vi "Channels.Inline.Write.Channel Block Descriptor (single).vi"(8 "error in (no error)":errorcluster, 10 "Values Array in":dbl[](array[numeric]), 11 "Channel Block Descriptor":T1) -> (0 "error out":errorcluster, 2 "Values Array out":dbl[](array[numeric]), 3 "Channel Block Descriptor dup":T1)   [LabVIEW 2016, in "VeriStand Data.lvlib"]
doc: "Writes the contents of <B>Values Array</B> to the memory location specified by <B>Channel Block Descriptor</B>."
uses:
  VeriStand Data.lvlib
  Typedefs/Typedefs.Block Descriptor.Channel Block.ctl
  Typedefs/Typedefs.Block Descriptor.ctl
  Memory Management/Memory Management.Handle Return.vi
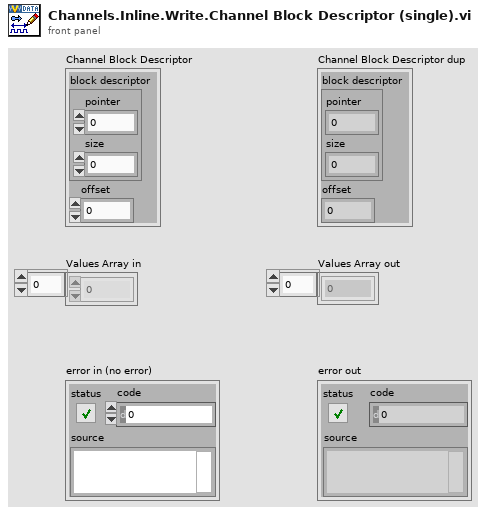
[diagram p1: front panel]
types:
  T1 = typedef "VeriStand Data.lvlib/Typedefs.Block Descriptor.Channel Block.ctl" = cluster{"block descriptor":T2, "offset":u64}
  T2 = typedef "VeriStand Data.lvlib/Typedefs.Block Descriptor.ctl" = cluster{"pointer":u64, "size":i64}
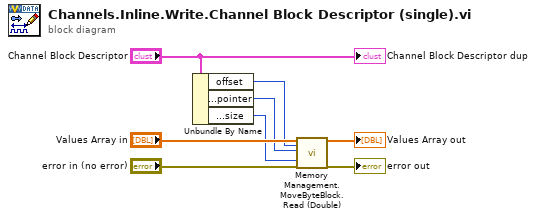
[diagram p0: block diagram]
diagram:
  n1 = Unbundle By Name("Channel Block Descriptor") -> ("offset"=w2:u64, "block descriptor.pointer"=w1:u64, "block descriptor.size"=w3:i64)
  n2 = call "Memory Management.MoveByteBlock.Read (Double).vi"("src in"="Values Array in", "src offset (0)"=w2, "dst ptr in"=w1, "size"=w3, "error in (no error)"="error in (no error)") -> ("src out"=→"Values Array out":dbl[], "error out"=→"error out":errorcluster)  [unwired: 9 in, 4 out]
  "Channel Block Descriptor dup" <- "Channel Block Descriptor"
